vi "SA_Best_Solution.vi"(8 "error in (no error)":errorcluster, 10 "GA.lvclass":refnum<class "GA.lvclass">, 11 "OSSP_Problem in":refnum<class "OSSP_Problem.lvclass">) -> (0 "error out":errorcluster, 2 "OSSP_Problem out":refnum<class "OSSP_Problem.lvclass">, 3 "GA out":refnum<class "GA.lvclass">)   [LabVIEW 2013]
uses:
  Classes/GA.lvclass
  Classes/OSSP_Problem.lvclass
  Classes/SA.lvclass
  SA/Controls/States_SA.ctl
  Classes/GA_Class/Controls/Solution_GA.ctl
  Classes/OSSP_Problem.lvclass/OSSP_Problem.ctl
  Classes/GA.lvclass/GA.ctl
  Classes/SA.lvclass/SA.ctl
  Classes/SA_Class/Controls/Solution_SA.ctl
  Classes/GanntChart_Class/Operation to Machine Job Tuple.vi
  Classes/GanntChart_Class/Check Other Machines for Schedule Time.vi
  Classes/GanntChart_Class/Schedule Job.vi
  Classes/GanntChart_Class/Find Gaps on Particular Machine.vi
  Classes/GanntChart_Class/Increment Number of Jobs on Machine.vi
  Classes/GanntChart_Class/Find Job On Other Machines.vi
  Classes/GanntChart.lvclass
panel:
  out "Best Tardiness/Makespan":u16
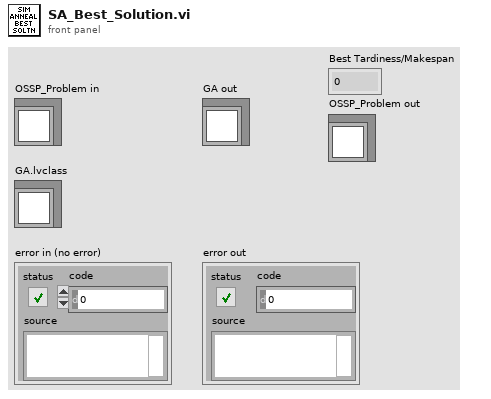
[diagram p1: front panel]
types:
  T1 = typedef "Solution_GA.ctl" = cluster{"Schedule":u16[], "Fitness":u16, "Fitness Valid?":bool}
  T2 = typedef "States_SA.ctl" = enum16{"Init", "Read Problem", "Sort Problem", "Generate and Evaluate Current Solution", "Perturb Cur Solution and Eval New Solution", "Make Decision", "Keep Track of Best Solution", "Cool", "Output Final Solution", "Stop"}
  T3 = typedef "Scheduler Type.ctl" = enum16{"Non Delay Scheduler", "GT Active Scheduler", "My Scheduler"}
  T4 = typedef "Objective.ctl" = enum16{"Makespan", "Total Tardiness"}
  T5 = typedef "Solution_SA.ctl" = cluster{"Schedule":u16[], "Fitness":i16}
  T6 = typedef "GanntChart_Element.ctl" = cluster{"Operation Number":i32, "Job Number":i32, "Start Time":i32, "Procesing Time":u16, "End Time":i32}
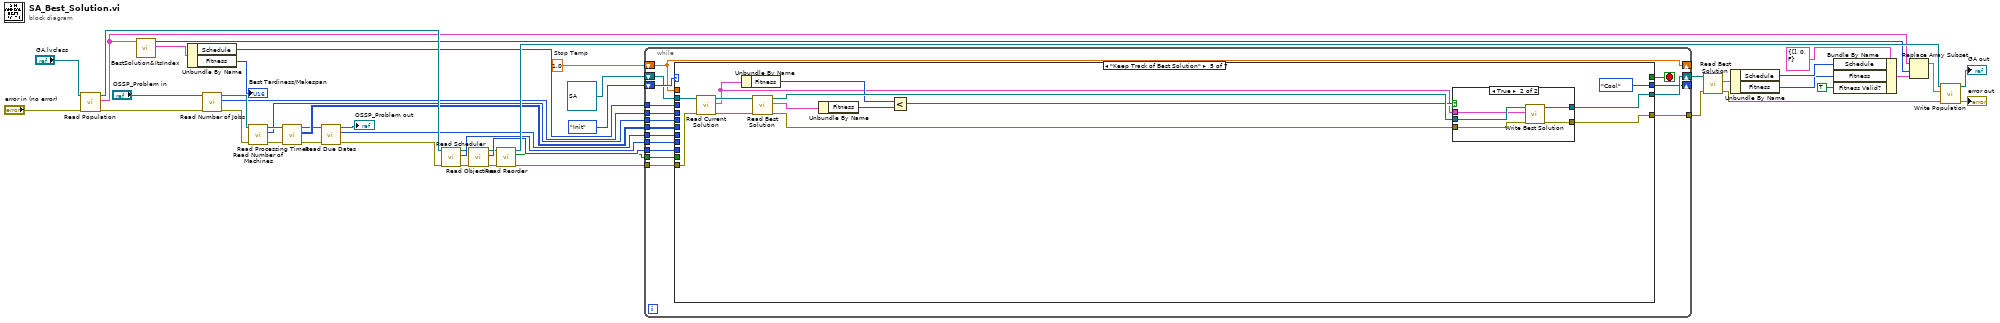
[diagram p0: block diagram]
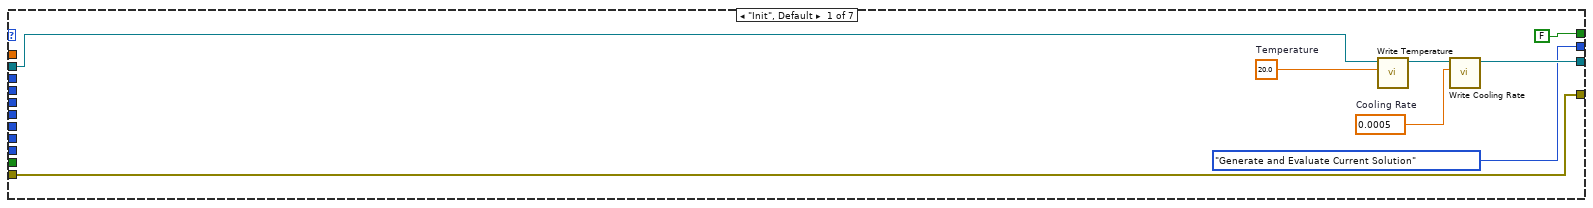
[diagram p2: hidden frame]
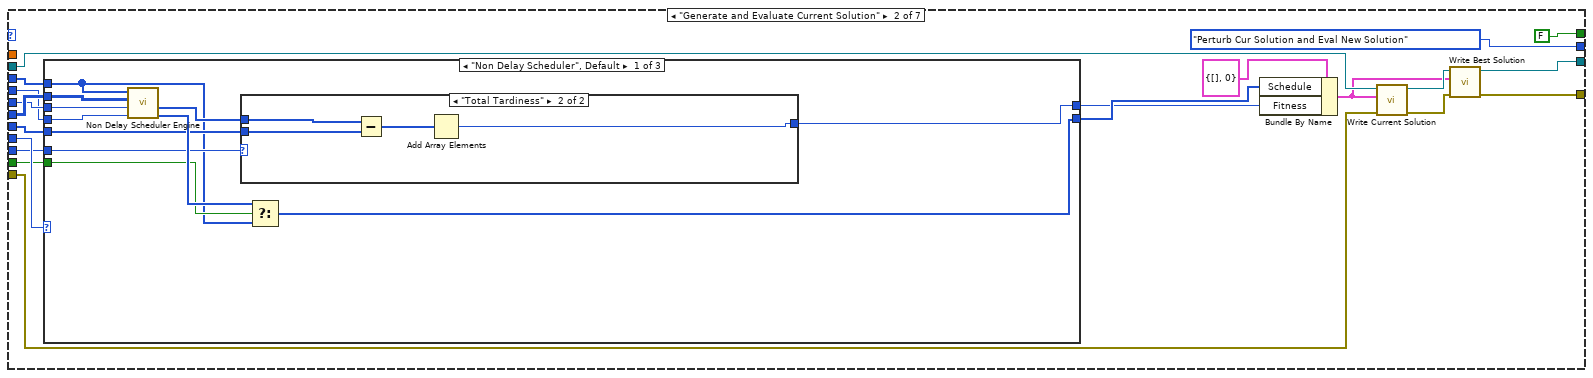
[diagram p3: hidden frame]
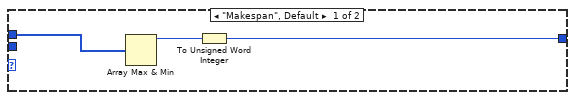
[diagram p4: hidden frame]
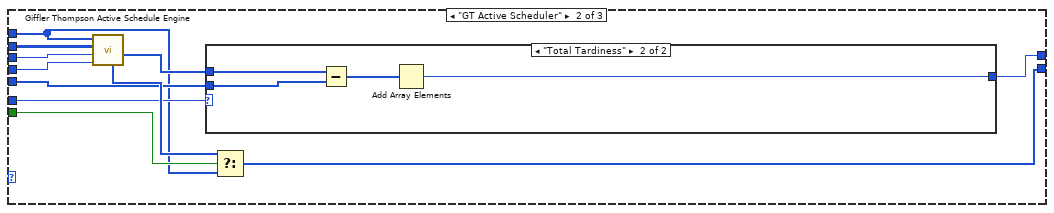
[diagram p5: hidden frame]
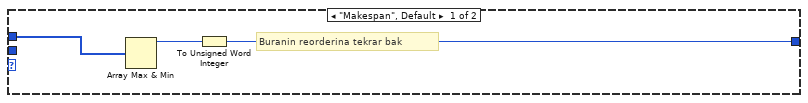
[diagram p6: hidden frame]
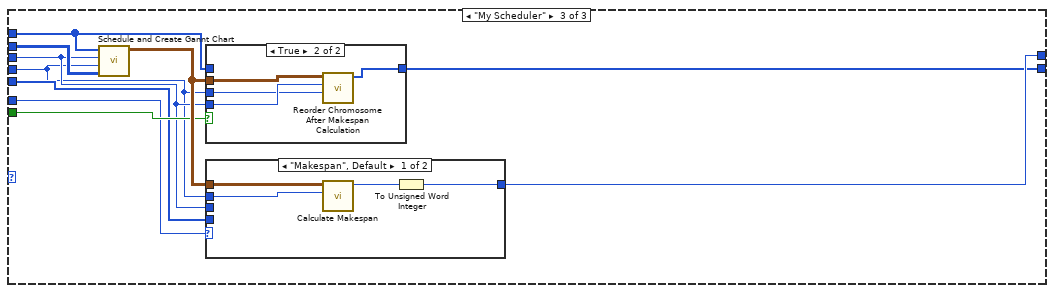
[diagram p7: hidden frame]
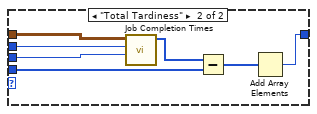
[diagram p9: hidden frame]
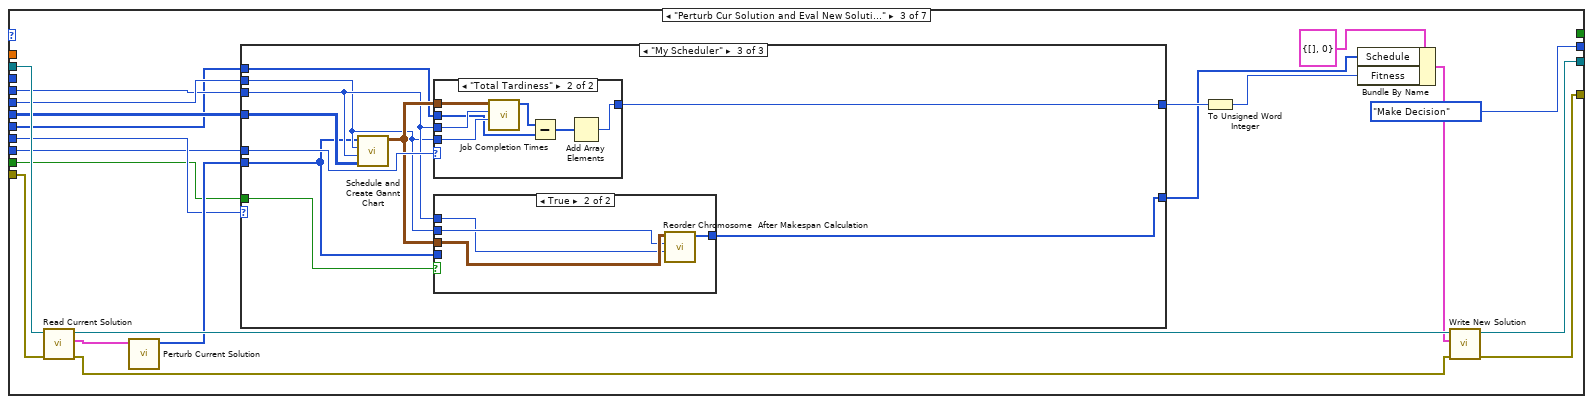
[diagram p10: hidden frame]
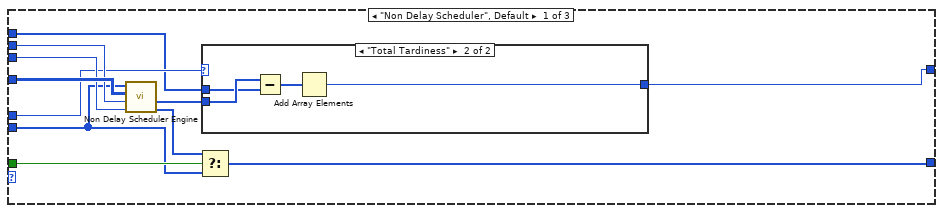
[diagram p11: hidden frame]
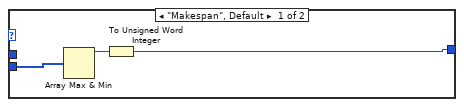
[diagram p12: hidden frame]
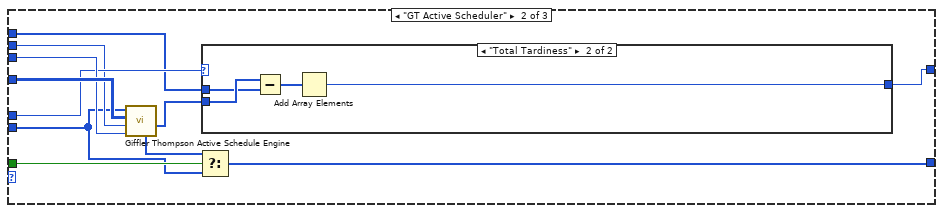
[diagram p13: hidden frame]
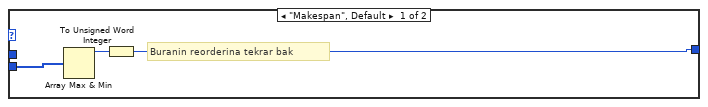
[diagram p14: hidden frame]
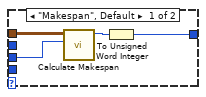
[diagram p16: hidden frame]
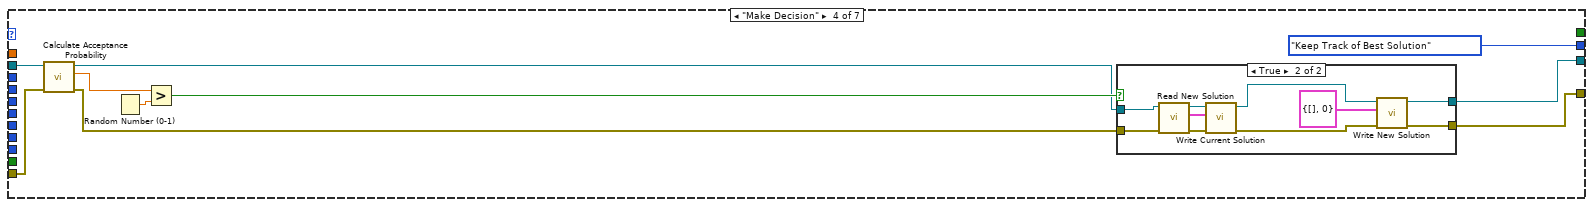
[diagram p17: hidden frame]
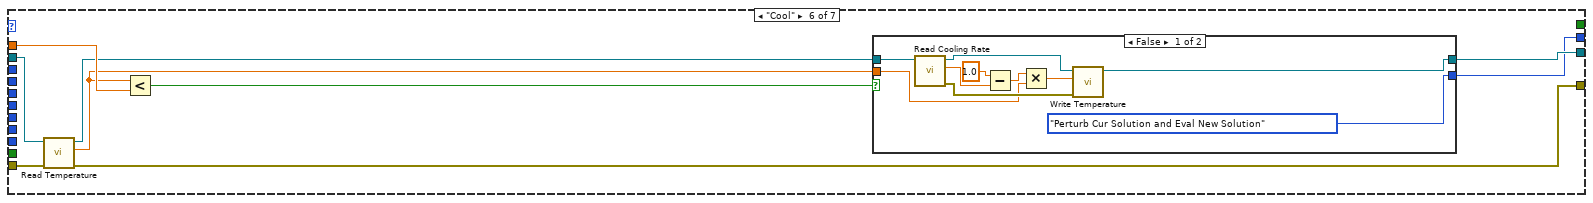
[diagram p20: hidden frame]
diagram:
  w31 = 1.0  # Stop Temp
  n1 = call-dynamic "Read Population.vi"("error in (no error)"="error in (no error)", "GA in"="GA.lvclass") -> ("error out"=w39:errorcluster, "Population"=w12:T1[], "GA out"=w40:refnum<class "GA.lvclass">)  [unwired: 7 in]
  n2 = call "BestSolution&ItsIndex.vi"("Population"=w12) -> ("Best Solution In the Population"=w14:T1, "Best Solution Index for Replace"=w11:i32)  [unwired: 9 in]
  n3 = Unbundle By Name(w14) -> ("Schedule"=w6:u16[], "Fitness"=→"Best Tardiness/Makespan":u16)
  n4 = call-dynamic "Read Number of Jobs.vi"("error in (no error)"=w39, "OSSP_Problem in"="OSSP_Problem in") -> ("error out"=w28:errorcluster, "Number of Jobs"=w34:i32, "OSSP_Problem out"=w36:refnum<class "OSSP_Problem.lvclass">)  [unwired: 7 in]
  n5 = call-dynamic "Read Number of Machines.vi"("error in (no error)"=w28, "OSSP_Problem in"=w36) -> ("error out"=w27:errorcluster, "Number of Machines"=w33:i32, "OSSP_Problem out"=w35:refnum<class "OSSP_Problem.lvclass">)  [unwired: 7 in]
  n6 = call-dynamic "Read Processing Times.vi"("error in (no error)"=w27, "OSSP_Problem in"=w35) -> ("error out"=w26:errorcluster, "Processing Times"=w32:u16[][], "OSSP_Problem out"=w25:refnum<class "OSSP_Problem.lvclass">)  [unwired: 7 in]
  n7 = call "Read Due Dates.vi"("error in (no error)"=w26, "OSSP_Problem in"=w25) -> ("error out"=w23:errorcluster, "Due Dates"=w24:u16[], "OSSP_Problem out"=→"OSSP_Problem out":refnum<class "OSSP_Problem.lvclass">)  [unwired: 7 in]
  n8 = call "Read Scheduler.vi"("error in (no error)"=w23, "GA in"=w40) -> ("error out"=w21:errorcluster, "Scheduler"=w22:T3, "GA out"=w20:refnum<class "GA.lvclass">)  [unwired: 7 in]
  n9 = call "Read Objective .vi"("error in (no error)"=w21, "GA in"=w20) -> ("error out"=w18:errorcluster, "Objective"=w19:T4, "GA out"=w15:refnum<class "GA.lvclass">)  [unwired: 7 in]
  n10 = call "Read Reorder.vi"("error in (no error)"=w18, "GA in"=w15) -> ("error out"=w17:errorcluster, "Reorder"=w16:bool, "GA out"=w41:refnum<class "GA.lvclass">)  [unwired: 7 in]
  n11 = while {
    tunnel: w6 -> [w60]
    shift-right: [w55] -> _
    shift-left: States_SA."Init" ("States") -> [w62]
    tunnel: w34 -> [w59]
    tunnel: w33 -> [w58]
    tunnel: w32 -> [w57]
    shift-right: [w56] -> w30
    shift-left: refnum<class "SA.lvclass"> refnum ("SA.lvclass") -> [w61]
    shift-right: [w54] -> _
    shift-left: w31 -> [w54]
    tunnel: [w52] -> w13
    tunnel: w17 -> [w51]
    tunnel: w24 -> [w50]
    tunnel: w22 -> [w49]
    tunnel: w19 -> [w48]
    tunnel: w16 -> [w47]
    stop <- w53 stop-if-true
    n12 = case shown="\"Keep Track of Best Solution\"" w62 {
      tunnel: w61 -> [w70 w90 w173 w245 w271 w287 w302]
      tunnel: w60 -> [_ w80 _ _ _ _ _]
      tunnel: w59 -> [_ w77 w167 _ _ _ _]
      tunnel: w58 -> [_ w78 w168 _ _ _ _]
      tunnel: w57 -> [_ w79 w166 _ _ _ _]
      tunnel: [w66 w85 w164 w244 w270 w282 w302] -> w56
      tunnel: [States_SA."Generate and Evaluate Current Solution" ("States") States_SA."Perturb Cur Solution and Eval New Solution" ("States") States_SA."Make Decision" ("States") States_SA."Keep Track of Best Solution" States_SA."Cool" w281 States_SA."Stop"] -> w55
      tunnel: w54 -> [_ _ _ _ _ w286 _]
      tunnel: [FALSE FALSE _ _ _ _ TRUE] -> w53
      tunnel: [w64 w71 w160 w236 w258 w279 w300] -> w52
      tunnel: w51 -> [w64 w72 w154 w238 w260 w280 w300]
      tunnel: w50 -> [_ w75 w157 _ _ _ _]
      tunnel: w49 -> [_ w83 w156 _ _ _ _]
      tunnel: w48 -> [_ w82 w155 _ _ _ _]
      tunnel: w47 -> [_ w81 w153 _ _ _ _]
      frame "Init", Default {
        w67 = 0.0005  # Cooling Rate
        w68 = 20.0  # Temperature
        n13 = call "Write Temperature.vi"("Temperature"=w68, "SA in"=w70) -> ("SA out"=w69:refnum<class "SA.lvclass">)  [unwired: 8 in, 1 out]
        n14 = call "Write Cooling Rate.vi"("Cooling Rate"=w67, "SA in"=w69) -> ("SA out"=w66:refnum<class "SA.lvclass">)  [unwired: 8 in, 1 out]
      }
      frame "Generate and Evaluate Current Solution" {
        n15 = case shown="\"Non Delay Scheduler\", Default" w83 {
          tunnel: [w97 w115 w136] -> w74
          tunnel: [w98 w116 w134] -> w76
          tunnel: w80 -> [w91 w109 w127]
          tunnel: w81 -> [w99 w119 w133]
          tunnel: w82 -> [w96 w112 w130]
          tunnel: w79 -> [w95 w114 w132]
          tunnel: w78 -> [w94 w111 w129]
          tunnel: w77 -> [w93 w110 w128]
          tunnel: w75 -> [w92 w113 w131]
          frame "Non Delay Scheduler", Default {
            n16 = call "Non Delay Scheduler Engine.vi"("Number of  Jobs"=w93, "Number of Machines"=w94, "Processing Times"=w95, "Schedule"=w91) -> ("Scheduled Jobs Order"=w100:u16[], "Job Completion Times"=w101:u16[])  [unwired: 3 in, 3 out]
            n17 = case shown="\"Total Tardiness\"" w96 {
              tunnel: w101 -> [w104 w108]
              tunnel: [w102 w105] -> w97
              tunnel: w92 -> [_ w107]
              frame "Makespan", Default {
                n18 = Array Max & Min(array=w104) -> (max value=w103:u16)  [unwired: 3 out]
                n19 = To Unsigned Word Integer(number=w103) -> (unsigned 16bit integer=w102:u16)
              }
              frame "Total Tardiness" {
                n20 = Subtract(x=w108, y=w107) -> (x-y=w106:u16[])
                n21 = Add Array Elements(numeric array=w106) -> (sum=w105:u16)
              }
            }
            n22 = Select(t=w100, s=w99, f=w91) -> (s? t:f=w98:u16[])
          }
          frame "GT Active Scheduler" {
            n23 = call "Giffler Thompson Active Schedule Engine.vi"("Number of  Jobs"=w110, "Number of Machines"=w111, "Processing Times"=w114, "Schedule In"=w109) -> ("Job Completion Times"=w117:u16[], "Schedule Order"=w118:u16[])  [unwired: 3 in, 3 out]
            n24 = case shown="\"Total Tardiness\"" w112 {
              tunnel: w117 -> [w122 w126]
              tunnel: [w120 w123] -> w115
              tunnel: w113 -> [_ w125]
              frame "Makespan", Default {
                # "Buranin reorderina tekrar bak"
                n25 = Array Max & Min(array=w122) -> (max value=w121:u16)  [unwired: 3 out]
                n26 = To Unsigned Word Integer(number=w121) -> (unsigned 16bit integer=w120:u16)
              }
              frame "Total Tardiness" {
                n27 = Subtract(x=w126, y=w125) -> (x-y=w124:u16[])
                n28 = Add Array Elements(numeric array=w124) -> (sum=w123:u16)
              }
            }
            n29 = Select(t=w118, s=w119, f=w109) -> (s? t:f=w116:u16[])
          }
          frame "My Scheduler" {
            n30 = call "Schedule and Create Gannt Chart.vi"("Processing Times (Rows Mach.Cols Jobs)"=w132, "Number of Jobs"=w128, "Number of Machines"=w129, "Schedule"=w127) -> ("Gannt Chart Out"=w135:T6[][])  [unwired: 6 in, 1 out]
            n31 = case shown="True" w133 {
              tunnel: w135 -> [_ w141]
              tunnel: [w137 w140] -> w134
              tunnel: w129 -> [_ w139]
              tunnel: w128 -> [_ w138]
              tunnel: w127 -> [w137 _]
              frame False {
              }
              frame True {
                n32 = call "Reorder Chromosome  After Makespan Calculation.vi"("Number Of  Jobs"=w138, "Number Of Machines"=w139, "Gannt Chart In"=w141) -> ("Reordered Chromosome"=w140:u16[])  [unwired: 8 in]
              }
            }
            n33 = case shown="\"Makespan\", Default" w130 {
              tunnel: w135 -> [w145 w150]
              tunnel: [w143 w149] -> w136
              tunnel: w131 -> [_ w148]
              tunnel: w128 -> [w142 w147]
              tunnel: w129 -> [_ w146]
              frame "Makespan", Default {
                n34 = call "Calculate Makespan.vi"("Number of Jobs"=w142, "Gannt Chart In"=w145) -> ("Makespan"=w144:i32)  [unwired: 9 in]
                n35 = To Unsigned Word Integer(number=w144) -> (unsigned 16bit integer=w143:u16)
              }
              frame "Total Tardiness" {
                n36 = call "Job Completion Times.vi"("Number Of Machines"=w146, "Number Of Jobs"=w147, "Gannt Chart In"=w150) -> ("Job Completion Times"=w152:u16[])  [unwired: 8 in]
                n37 = Subtract(x=w152, y=w148) -> (x-y=w151:u16[])
                n38 = Add Array Elements(numeric array=w151) -> (sum=w149:u16)
              }
            }
          }
        }
        n39 = Bundle By Name(cluster=T5 {"Schedule"=[], "Fitness"=0} ("Solution"), "Schedule"=w76, "Fitness"=w74) -> (w84:T5)
        n40 = call "Write Current Solution.vi"("error in (no error)"=w72, "Solution"=w84, "SA in"=w90) -> ("error out"=w73:errorcluster, "SA out"=w86:refnum<class "SA.lvclass">)  [unwired: 7 in]
        n41 = call "Write Best Solution.vi"("error in (no error)"=w73, "Solution"=w84, "SA in"=w86) -> ("error out"=w71:errorcluster, "SA out"=w85:refnum<class "SA.lvclass">)  [unwired: 7 in]
      }
      frame "Perturb Cur Solution and Eval New Solution" {
        n42 = call "Read Current Solution.vi"("error in (no error)"=w154, "SA in"=w173) -> ("error out"=w161:errorcluster, "Solution"=w172:T5, "SA out"=w171:refnum<class "SA.lvclass">)  [unwired: 7 in]
        n43 = call "Perturb Current Solution.vi"("Solution"=w172) -> ("Schedule"=w169:u16[])  [unwired: 10 in]
        n44 = case shown="\"My Scheduler\"" w156 {
          tunnel: w169 -> [w178 w194 w210]
          tunnel: w168 -> [w180 w196 w213]
          tunnel: w167 -> [w181 w198 w215]
          tunnel: w166 -> [w182 w202 w219]
          tunnel: [w174 w192 w218] -> w159
          tunnel: w155 -> [w176 w197 w217]
          tunnel: [w177 w193 w214] -> w158
          tunnel: w157 -> [w175 w195 w212]
          tunnel: w153 -> [w179 w201 w211]
          frame "Non Delay Scheduler", Default {
            n45 = call "Non Delay Scheduler Engine.vi"("Number of  Jobs"=w181, "Number of Machines"=w180, "Processing Times"=w182, "Schedule"=w178) -> ("Scheduled Jobs Order"=w183:u16[], "Job Completion Times"=w184:u16[])  [unwired: 3 in, 3 out]
            n46 = Select(t=w183, s=w179, f=w178) -> (s? t:f=w177:u16[])
            n47 = case shown="\"Total Tardiness\"" w176 {
              tunnel: w184 -> [w187 w191]
              tunnel: [w185 w188] -> w174
              tunnel: w175 -> [_ w190]
              frame "Makespan", Default {
                n48 = Array Max & Min(array=w187) -> (max value=w186:u16)  [unwired: 3 out]
                n49 = To Unsigned Word Integer(number=w186) -> (unsigned 16bit integer=w185:u16)
              }
              frame "Total Tardiness" {
                n50 = Subtract(x=w191, y=w190) -> (x-y=w189:u16[])
                n51 = Add Array Elements(numeric array=w189) -> (sum=w188:u16)
              }
            }
          }
          frame "GT Active Scheduler" {
            n52 = call "Giffler Thompson Active Schedule Engine.vi"("Number of  Jobs"=w198, "Number of Machines"=w196, "Processing Times"=w202, "Schedule In"=w194) -> ("Job Completion Times"=w199:u16[], "Schedule Order"=w200:u16[])  [unwired: 3 in, 3 out]
            n53 = Select(t=w200, s=w201, f=w194) -> (s? t:f=w193:u16[])
            n54 = case shown="\"Total Tardiness\"" w197 {
              tunnel: w199 -> [w205 w209]
              tunnel: [w203 w206] -> w192
              tunnel: w195 -> [_ w208]
              frame "Makespan", Default {
                # "Buranin reorderina tekrar bak"
                n55 = Array Max & Min(array=w205) -> (max value=w204:u16)  [unwired: 3 out]
                n56 = To Unsigned Word Integer(number=w204) -> (unsigned 16bit integer=w203:u16)
              }
              frame "Total Tardiness" {
                n57 = Subtract(x=w209, y=w208) -> (x-y=w207:u16[])
                n58 = Add Array Elements(numeric array=w207) -> (sum=w206:u16)
              }
            }
          }
          frame "My Scheduler" {
            n59 = call "Schedule and Create Gannt Chart.vi"("Processing Times (Rows Mach.Cols Jobs)"=w219, "Number of Jobs"=w215, "Number of Machines"=w213, "Schedule"=w210) -> ("Gannt Chart Out"=w216:T6[][])  [unwired: 6 in, 1 out]
            n60 = case shown="\"Total Tardiness\"" w217 {
              tunnel: w216 -> [w228 w233]
              tunnel: [w225 w229] -> w218
              tunnel: w215 -> [w227 w232]
              tunnel: w213 -> [_ w231]
              tunnel: w212 -> [_ w230]
              frame "Makespan", Default {
                n61 = call "Calculate Makespan.vi"("Number of Jobs"=w227, "Gannt Chart In"=w228) -> ("Makespan"=w226:i32)  [unwired: 9 in]
                n62 = To Unsigned Word Integer(number=w226) -> (unsigned 16bit integer=w225:u16)
              }
              frame "Total Tardiness" {
                n63 = call "Job Completion Times.vi"("Number Of Machines"=w231, "Number Of Jobs"=w232, "Gannt Chart In"=w233) -> ("Job Completion Times"=w235:u16[])  [unwired: 8 in]
                n64 = Subtract(x=w235, y=w230) -> (x-y=w234:u16[])
                n65 = Add Array Elements(numeric array=w234) -> (sum=w229:u16)
              }
            }
            n66 = case shown="True" w211 {
              tunnel: w216 -> [_ w224]
              tunnel: w213 -> [_ w223]
              tunnel: w215 -> [_ w222]
              tunnel: [w220 w221] -> w214
              tunnel: w210 -> [w220 _]
              frame False {
              }
              frame True {
                n67 = call "Reorder Chromosome  After Makespan Calculation.vi"("Number Of  Jobs"=w222, "Number Of Machines"=w223, "Gannt Chart In"=w224) -> ("Reordered Chromosome"=w221:u16[])  [unwired: 8 in]
              }
            }
          }
        }
        n68 = To Unsigned Word Integer(number=w159) -> (unsigned 16bit integer=w162:u16)
        n69 = Bundle By Name(cluster=T5 {"Schedule"=[], "Fitness"=0} ("Solution"), "Schedule"=w158, "Fitness"=w162) -> (w165:T5)
        n70 = call "Write New Solution.vi"("error in (no error)"=w161, "Solution"=w165, "SA in"=w171) -> ("error out"=w160:errorcluster, "SA out"=w164:refnum<class "SA.lvclass">)  [unwired: 7 in]
      }
      frame "Make Decision" {
        n71 = call "Calculate Acceptance Probability.vi"("error in (no error)"=w238, "SA in"=w245) -> ("error out"=w237:errorcluster, "Acceptance Probability"=w242:dbl, "SA out"=w239:refnum<class "SA.lvclass">)  [unwired: 7 in]
        n72 = Random Number (0-1)() -> (number: 0 to 1=w241:dbl)
        n73 = Greater?(x=w242, y=w241) -> (0:w240:bool)
        n74 = case shown="True" w240 {
          tunnel: w239 -> [w247 w257]
          tunnel: [w247 w251] -> w244
          tunnel: w237 -> [w246 w250]
          tunnel: [w246 w249] -> w236
          frame False {
          }
          frame True {
            n75 = call "Read New Solution.vi"("error in (no error)"=w250, "SA in"=w257) -> ("error out"=w256:errorcluster, "Solution"=w254:T5, "SA out"=w255:refnum<class "SA.lvclass">)  [unwired: 7 in]
            n76 = call "Write Current Solution.vi"("error in (no error)"=w256, "Solution"=w254, "SA in"=w255) -> ("error out"=w252:errorcluster, "SA out"=w253:refnum<class "SA.lvclass">)  [unwired: 7 in]
            n77 = call "Write New Solution.vi"("error in (no error)"=w252, "Solution"=T5 {"Schedule"=[], "Fitness"=0}, "SA in"=w253) -> ("error out"=w249:errorcluster, "SA out"=w251:refnum<class "SA.lvclass">)  [unwired: 7 in]
          }
        }
      }
      frame "Keep Track of Best Solution" {
        n78 = call "Read Current Solution.vi"("error in (no error)"=w260, "SA in"=w271) -> ("error out"=w261:errorcluster, "Solution"=w263:T5, "SA out"=w269:refnum<class "SA.lvclass">)  [unwired: 7 in]
        n79 = Unbundle By Name(w263) -> ("Fitness"=w267:i16)
        n80 = call "Read Best Solution.vi"("error in (no error)"=w261, "SA in"=w269) -> ("error out"=w259:errorcluster, "Solution"=w266:T5, "SA out"=w268:refnum<class "SA.lvclass">)  [unwired: 7 in]
        n81 = Unbundle By Name(w266) -> ("Fitness"=w265:i16)
        n82 = Less?(x=w267, y=w265) -> (x < y?=w264:bool)
        n83 = case shown="True" w264 {
          tunnel: w268 -> [w273 w278]
          tunnel: [w273 w277] -> w270
          tunnel: w263 -> [_ w276]
          tunnel: w259 -> [w272 w275]
          tunnel: [w272 w274] -> w258
          frame False {
          }
          frame True {
            n84 = call "Write Best Solution.vi"("error in (no error)"=w275, "Solution"=w276, "SA in"=w278) -> ("error out"=w274:errorcluster, "SA out"=w277:refnum<class "SA.lvclass">)  [unwired: 7 in]
          }
        }
      }
      frame "Cool" {
        n85 = call "Read Temperature.vi"("error in (no error)"=w280, "SA in"=w287) -> ("error out"=w279:errorcluster, "Temperature"=w283:dbl, "SA out"=w284:refnum<class "SA.lvclass">)  [unwired: 7 in]
        n86 = Less?(x=w283, y=w286) -> (x < y?=w285:bool)
        n87 = case shown="False" w285 {
          tunnel: [States_SA."Perturb Cur Solution and Eval New Solution" ("f") States_SA."Stop"] -> w281
          tunnel: w284 -> [w295 w298]
          tunnel: [w296 w298] -> w282
          tunnel: w283 -> [w288 _]
          frame False {
            n88 = call "Read Cooling Rate.vi"("SA in"=w295) -> ("error out"=w293:errorcluster, "Cooling Rate"=w291:dbl, "SA out"=w294:refnum<class "SA.lvclass">)  [unwired: 8 in]
            n89 = Subtract(x=1.0, y=w291) -> (x-y=w290:dbl)
            n90 = Multiply(x=w290, y=w288) -> (x*y=w289:dbl)
            n91 = call "Write Temperature.vi"("error in (no error)"=w293, "Temperature"=w289, "SA in"=w294) -> ("SA out"=w296:refnum<class "SA.lvclass">)  [unwired: 7 in, 1 out]
          }
          frame True {
          }
        }
      }
      frame "Stop" {
      }
    }
  }
  n92 = call "Read Best Solution.vi"("error in (no error)"=w13, "SA in"=w30) -> ("error out"=w4:errorcluster, "Solution"=w29:T5)  [unwired: 7 in, 1 out]
  n93 = Unbundle By Name(w29) -> ("Schedule"=w2:u16[], "Fitness"=w1:i16)
  n94 = Bundle By Name(cluster=T1 {"Schedule"=[], "Fitness"=0, "Fitness Valid?"=FALSE} ("new element/subarray"), "Schedule"=w2, "Fitness"=w1, "Fitness Valid?"=TRUE) -> (w10:T1)
  n95 = Replace Array Subset(array=w12, new element=w10, index=w11) -> (w9:T1[])
  n96 = call "Write Population.vi"("error in (no error)"=w4, "Population"=w9, "GA in"=w41) -> ("error out"=→"error out":errorcluster, "GA out"=→"GA out":refnum<class "GA.lvclass">)  [unwired: 7 in]
